vi "DAQNavi Read (Digital 1D Wfm NChan 1Samp).vi"(8 "error in (no error)":errorcluster, 10 "timeout":dbl=10.0 format="%0.2f", 11 "task in":i32) -> (0 "error out":errorcluster, 2 "data":digitalwaveform[](array[waveform]), 3 "task out":i32)   [LabVIEW 2020]
uses:
  DAQNavi_LV.dll
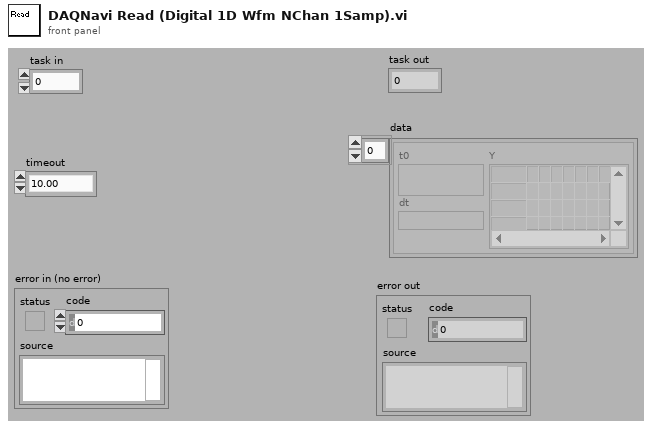
[diagram p1: front panel]
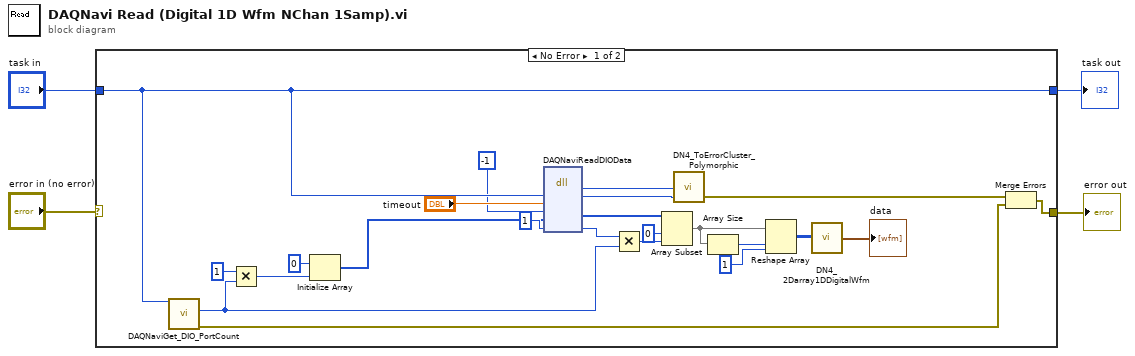
[diagram p0: block diagram]
diagram:
  n1 = case shown="No Error" "error in (no error)" {
    selector: "error in (no error)" -> [_ w28]
    tunnel: "task in" -> [w21 w29]
    tunnel: [w21 w29] -> w2
    tunnel: [w18 w28] -> w1
    frame No Error {
      n2 = call "DAQNaviGet_DIO_PortCount.vi"("task in"=w21) -> ("error out"=w19:errorcluster, "port count"=w15:i32)  [unwired: 1 in, 8 out]
      n3 = Multiply(x=1 ("y"), y=w15) -> (x*y=w22:i32)
      n4 = Initialize Array(u8 0 ("element"), w22) -> (w13:u8[])
      n5 = dll-call lib="DAQNavi_LV.dll" fn="DAQNaviReadDIOData"("taskID"=w21, "timeout"="timeout", "portBit"=-1, "portData"=w13, "samples"=1) -> ("return type"=w24:i32, "taskID"=w6:i32, "portData"=w12:u8[], "samples"=w16:i32)  [unwired: 5 in, 2 out]
      n6 = Multiply(x=w16, y=w15) -> (x*y=w14:i32)
      n7 = Array Subset(array=w12, index=0, length=w14) -> (w10:u8[])
      n8 = call "DN4_ToErrorCluster_Polymorphic.vi"("task id"=w6, "error code"=w24) -> ("error out"=w20:errorcluster)  [unwired: 3 out]
      n9 = Array Size(array=w10) -> (size(s)=w11:i32)
      n10 = Reshape Array(w10, w11, 1 ("dimension size")) -> (w8:u8[][])
      n11 = call "DN4_2Darray1DDigitalWfm.vi"("data"=w8) -> ("1D Wfm"=→"data":digitalwaveform[])
      n12 = Merge Errors(w20, w19) -> (w18:errorcluster)
    }
    frame Error {
    }
  }
  "task out" <- w2
  "error out" <- w1
